vi "HFRR ADV v011 new software.vi"() -> ()   [LabVIEW 2025] (continued)
            n1484 = Equal?(x=w2429, y=10) -> (x = y?=w2427:bool)
            n1485 = case shown="True" w2427 {
              frame False {
                n1486 = property on="ENTER THE NEW PASSWORD" class="Str"("Visible"=FALSE) -> ()  [unwired: 2 in, 2 out]
              }
              frame True {
                # "password"
                # "change password logic"
                n1487 = local read "ENTER CURRENT PASSWORD"() -> (w2446:string)
                n1488 = local read "dipl pwd"() -> (w2440:string)
                n1489 = String To Byte Array(string=w2446) -> (unsigned byte array=w2448:u8[])
                n1490 = String To Byte Array(string=w2440) -> (unsigned byte array=w2441:u8[])
                n1491 = Array Size(array=w2448) -> (size(s)=w2445:i32)
                n1492 = Array Size(array=w2441) -> (size(s)=w2443:i32)
                n1493 = for {
                  N: w2445 -> [_]
                  tunnel: w2448 -> [w2472]
                  tunnel: [w2470] -> w2449 mode=indexing
                  tunnel: w2445 -> [w2464]
                  i -> [w2465]
                  n1494 = Decrement(x=w2464) -> (x-1=w2462:i32)
                  n1495 = Equal?(x=w2465, y=w2462) -> (x = y?=w2463:bool)
                  n1496 = Index Array(array=w2472, index=w2465) -> (element=w2466:u8)
                  n1497 = Number To Decimal String(number=w2466) -> (decimal integer string=w2471:string)  [unwired: 1 in]
                  n1498 = Select(t="", s=w2463, f="\r") -> (s? t:f=w2468:string)
                  n1499 = Concatenate Strings(w2471, w2468) -> (w2470:string)
                }
                n1500 = for {
                  N: w2443 -> [_]
                  tunnel: w2441 -> [w2460]
                  tunnel: [w2458] -> w2442 mode=indexing
                  tunnel: w2443 -> [w2455]
                  i -> [w2456]
                  n1501 = Decrement(x=w2455) -> (x-1=w2454:i32)
                  n1502 = Equal?(x=w2456, y=w2454) -> (x = y?=w2453:bool)
                  n1503 = Index Array(array=w2460, index=w2456) -> (element=w2459:u8)
                  n1504 = Number To Decimal String(number=w2459) -> (decimal integer string=w2457:string)  [unwired: 1 in]
                  n1505 = Select(t="", s=w2453, f="\r") -> (s? t:f=w2450:string)
                  n1506 = Concatenate Strings(w2457, w2450) -> (w2458:string)
                }
                n1507 = local read "string"() -> (w2447:string)
                n1508 = Concatenate Strings(w2442) -> (w2436:string)
                n1509 = Concatenate Strings(w2447) -> (w2444:string)
                n1510 = Concatenate Strings(w2449) -> (w2437:string)
                n1511 = Equal?(x=w2437, y=w2444) -> (x = y?=w2439:bool)
                n1512 = Equal?(x=w2437, y=w2436) -> (x = y?=w2435:bool)
                n1513 = Or(x=w2439, y=w2435) -> (x .or. y?=w2438:bool)
                n1514 = case shown="True" w2438 {
                  frame False {
                  }
                  frame True {
                    n1515 = property on="ENTER THE NEW PASSWORD" class="Str"("Visible"=TRUE) -> ()  [unwired: 2 in, 2 out]
                  }
                }
              }
            }
          }
          frame #2 {
            n1516 = String To Byte Array(string="ENTER THE NEW PASSWORD") -> (unsigned byte array=w2475:u8[])
            n1517 = Search 1D Array(1D array=w2475, element=u8 10) -> (index of element=w2479:i32)  [unwired: 1 in]
            n1518 = Index Array(array=w2475, index=w2479) -> (element=w2477:u8)
            n1519 = Equal?(x=w2477, y=10) -> (x = y?=w2474:bool)
            n1520 = case shown="False" w2474 {
              frame False {
              }
              frame True {
                n1521 = local write "EDIT"(FALSE) -> ()
                n1522 = local write "SrvM CP"(FALSE) -> ()
                n1523 = local read "ENTER THE NEW PASSWORD"() -> (w2482:string)
                n1524 = String To Byte Array(string=w2482) -> (unsigned byte array=w2487:u8[])
                n1525 = Array Size(array=w2487) -> (size(s)=w2484:i32)
                n1526 = for {
                  N: w2484 -> [_]
                  tunnel: w2487 -> [w2500]
                  tunnel: [w2497] -> w2489 mode=indexing
                  tunnel: w2484 -> [w2492]
                  i -> [w2490]
                  n1527 = Decrement(x=w2492) -> (x-1=w2493:i32)
                  n1528 = Equal?(x=w2490, y=w2493) -> (x = y?=w2494:bool)
                  n1529 = Index Array(array=w2500, index=w2490) -> (element=w2499:u8)
                  n1530 = Number To Decimal String(number=w2499) -> (decimal integer string=w2498:string)  [unwired: 1 in]
                  n1531 = Select(t="", s=w2494, f="\r") -> (s? t:f=w2491:string)
                  n1532 = Concatenate Strings(w2498, w2491) -> (w2497:string)
                }
                n1533 = local read "file path"() -> (w2481:path)
                n1534 = Concatenate Strings(w2489) -> (w2483:string)
                n1535 = Delete(path (use dialog)=w2481) -> (deleted path=w2485:path)  [unwired: 4 in, 2 out]
                n1536 = call <vilib>:"Write Characters To File.vi"("append to file? (new file:F)"=FALSE, "character string"=w2483, "file path (dialog if empty)"=w2485) -> ()  [unwired: 2 in, 1 out]
              }
            }
          }
          frame #3 {
            n1537 = case shown="True" "SrvM CP" {
              frame False {
                w2503 = ""
                n1538 = local write "ENTER CURRENT PASSWORD"(w2503) -> ()
                n1539 = local write "ENTER THE NEW PASSWORD"(w2503) -> ()
                n1540 = property on="ENTER CURRENT PASSWORD" class="Str"("Visible"=FALSE) -> ()  [unwired: 2 in, 2 out]
              }
              frame True {
                n1541 = property on="ENTER THE NEW PASSWORD" class="Str"() -> ("Visible"=w2504:bool)  [unwired: 2 in, 2 out]
                n1542 = Not(x=w2504) -> (.not. x?=w2505:bool)
                n1543 = property on="ENTER CURRENT PASSWORD" class="Str"("Visible"=w2505) -> ()  [unwired: 2 in, 2 out]
              }
            }
          }
          frame #4 {
            n1544 = String To Byte Array(string="Password") -> (unsigned byte array=w2512:u8[])
            n1545 = Search 1D Array(1D array=w2512, element=u8 10) -> (index of element=w2510:i32)  [unwired: 1 in]
            n1546 = Index Array(array=w2512, index=w2510) -> (element=w2511:u8)
            n1547 = Equal?(x=w2511, y=10) -> (x = y?=w2507:bool)
            n1548 = case shown="True" w2507 {
              frame False {
              }
              frame True {
                # "password"
                # "password"
                n1549 = local read "Password"() -> (w2525:string)
                n1550 = String To Byte Array(string=w2525) -> (unsigned byte array=w2528:u8[])
                n1551 = String To Byte Array(string="@143$\n") -> (unsigned byte array=w2514:u8[])
                n1552 = Array Size(array=w2528) -> (size(s)=w2523:i32)
                n1553 = Array Size(array=w2514) -> (size(s)=w2519:i32)
                n1554 = for {
                  N: w2523 -> [_]
                  tunnel: w2528 -> [w2562]
                  tunnel: [w2560] -> w2529 mode=indexing
                  tunnel: w2523 -> [w2557]
                  i -> [w2558]
                  n1555 = Decrement(x=w2557) -> (x-1=w2556:i32)
                  n1556 = Index Array(array=w2562, index=w2558) -> (element=w2561:u8)
                  n1557 = Equal?(x=w2558, y=w2556) -> (x = y?=w2555:bool)
                  n1558 = Number To Decimal String(number=w2561) -> (decimal integer string=w2559:string)  [unwired: 1 in]
                  n1559 = Select(t="", s=w2555, f="\r") -> (s? t:f=w2552:string)
                  n1560 = Concatenate Strings(w2559, w2552) -> (w2560:string)
                }
                n1561 = for {
                  N: w2519 -> [_]
                  tunnel: w2514 -> [w2573]
                  tunnel: [w2571] -> w2517 mode=indexing
                  tunnel: w2519 -> [w2568]
                  i -> [w2569]
                  n1562 = Decrement(x=w2568) -> (x-1=w2567:i32)
                  n1563 = Index Array(array=w2573, index=w2569) -> (element=w2572:u8)
                  n1564 = Equal?(x=w2569, y=w2567) -> (x = y?=w2566:bool)
                  n1565 = Number To Decimal String(number=w2572) -> (decimal integer string=w2570:string)  [unwired: 1 in]
                  n1566 = Select(t="", s=w2566, f="\r") -> (s? t:f=w2563:string)
                  n1567 = Concatenate Strings(w2570, w2563) -> (w2571:string)
                }
                n1568 = local read "file path"() -> (w2513:path)
                n1569 = call <vilib>:"Read Characters From File.vi"("file path (dialog if empty)"=w2513) -> ("character string"=w2527:string)  [unwired: 5 in, 3 out]
                "string" <- w2527
                n1570 = flat-sequence {
                  tunnel: [w2530] -> w2524
                  frame #0 {
                    w2530 = ""
                    n1571 = local write "Password"(w2530) -> ()
                  }
                }
                n1572 = Concatenate Strings(w2517) -> (w2518:string)
                n1573 = Concatenate Strings(w2527) -> (w2526:string)
                n1574 = Concatenate Strings(w2529) -> (w2521:string)
                n1575 = Equal?(x=w2521, y=w2526) -> (x = y?=w2516:bool)
                n1576 = Equal?(x=w2521, y=w2518) -> (x = y?=w2522:bool)
                n1577 = Or(x=w2516, y=w2522) -> (x .or. y?=w2515:bool)
                "x = y?" <- w2515
                n1578 = case shown="True" w2515 {
                  selector: w2515 -> [w2532 _]
                  tunnel: w2524 -> [_ _]
                  frame False {
                    n1579 = And(x=w2532, y=TRUE ("Visible")) -> (x .and. y?=w2533:bool)
                    n1580 = property on="message" class="Str"("Visible"=w2533) -> ()  [unwired: 2 in, 2 out]
                  }
                  frame True {
                    n1581 = control-ref of="This VI"() -> (w2544:refnum<vi>)
                    n1582 = property class="VI"(reference=w2544) -> (reference out=w2535:refnum<vi>, error out=w2539:errorcluster, "Panel"=w2543:refnum<vi>)  [unwired: 1 in]
                    n1583 = property on="message" class="Str"("Visible"=FALSE) -> ()  [unwired: 2 in, 2 out]
                    n1584 = property class="Pnl"(reference=w2543, error in=w2539) -> (reference out=w2537:refnum<vi>, error out=w2540:errorcluster, "Panes[]"=w2542:refnum<vi>[])
                    n1585 = for {
                      tunnel: w2542 -> [w2551] mode=indexing
                      tunnel: T20."Always On" ("Horizontal Scrollbar Visibility") -> [w2550]
                      tunnel: w2540 -> [w2547]
                      tunnel: [w2546] -> w2538
                      n1586 = property class="Pane"(reference=w2551, error in=w2547, "HorizScrollbarVisibility"=w2550) -> (reference out=w2548:refnum<vi>, error out=w2549:errorcluster)
                      n1587 = Close Reference(reference=w2548, error in (no error)=w2549) -> (error out=w2546:errorcluster)
                    }
                    n1588 = Close Reference(reference=w2537, error in (no error)=w2538) -> (error out=w2536:errorcluster)
                    n1589 = Close Reference(reference=w2535, error in (no error)=w2536) -> (error out=→"error out 6":errorcluster)
                  }
                }
              }
            }
          }
        }
        n1590 = local read "x = y?"() -> (w2372:bool)
        n1591 = local read "HUMIDITY: 2"() -> (w2374:dbl)
        n1592 = local read "HUMIDITY:"() -> (w2373:dbl)
        n1593 = property on="Port 2 Error" class="Clust (strict)"("Visible"="EDIT") -> ()  [unwired: 2 in, 2 out]
        n1594 = property on="Port 1 Error" class="Clust (strict)"("Visible"="EDIT") -> ()  [unwired: 2 in, 2 out]
        n1595 = case shown="True" "SrvM CP 2" {
          frame False {
          }
          frame True {
            n1596 = local write "SrvM CP 2"(FALSE ("SrvM CP 2")) -> ()
            n1597 = local read "HUMIDITY: 2"() -> (w2413:dbl)
            n1598 = local read "TEMP INTERCEPT: 2"() -> (w2412:dbl)
            n1599 = local read "DISPLACEMENT : 4"() -> (w2416:dbl)
            n1600 = local read "TEMPERATURE : 2"() -> (w2415:dbl)
            n1601 = local read "STROKE GAIN : 2"() -> (w2417:dbl)
            n1602 = local read "FRIC. FORCE : 2"() -> (w2418:dbl)
            n1603 = local read "AIR TEMP INTERCEPT: 2"() -> (w2411:dbl)
            n1604 = local read "AIR TEMPERATURE : 2"() -> (w2414:dbl)
            n1605 = local write "HUMIDITY:"(w2413) -> ()
            n1606 = local write "AIR TEMP INTERCEPT:"(w2412) -> ()
            n1607 = local write "TEMPERATURE :"(w2415) -> ()
            n1608 = local write "FRIC. FORCE :"(w2418) -> ()
            n1609 = local write "STROKE GAIN :"(w2417) -> ()
            n1610 = local write "DISPLACEMENT :"(w2416) -> ()
            n1611 = local write "AIR TEMPERATURE :"(w2414) -> ()
            n1612 = local write "TEMP INTERCEPT:"(w2411) -> ()
          }
        }
        n1613 = Or(x="SAVE", y=w2366) -> (x .or. y?=w2367:bool)
        n1614 = And(x="EDIT", y=w2372) -> (x .and. y?=w2370:bool)
        n1615 = local read "DISPLACEMENT : 4"() -> (w2383:dbl)
        n1616 = local read "TEMPERATURE : 2"() -> (w2381:dbl)
        n1617 = local read "STROKE GAIN : 2"() -> (w2387:dbl)
        n1618 = local read "DISPLACEMENT :"() -> (w2382:dbl)
        n1619 = local read "FRIC. FORCE : 2"() -> (w2390:dbl)
        n1620 = local read "TEMPERATURE :"() -> (w2379:dbl)
        n1621 = local read "STROKE GAIN :"() -> (w2386:dbl)
        n1622 = local read "FRIC. FORCE :"() -> (w2389:dbl)
        n1623 = case shown="True" w2370 {
          tunnel: [u8 2 ("Disabled") u8 0 ("Disabled")] -> w2369
          tunnel: [w2734 TRUE ("Visible")] -> w2368
          frame False {
            w2734 = FALSE ("Visible")
            n1624 = local write "EDIT 2"(w2734) -> ()
          }
          frame True {
          }
        }
        n1625 = case shown="True" w2367 {
          frame False {
          }
          frame True {
            n1626 = stacked-sequence {
              seq-local: [w2582 _ _] -> [_ w2729 _]
              frame #0 {
                (unwired) i16 5 ("precision (6)")
                # "[CH1]    - FF\n[CH2]   - TEMPERATURE\n[CH3]    - Humidity\n[CH4]    - AIR TEMP\n[CH5]\\- Visa Uno\n[CH6] \\- Visa Due\n[CH7]  \\- file path\n[CH8]   - Displacement Gain\n[CHA]   - Stroke Gain\n[CHB]   - Stroke PID Gain\n[CHC]   -Language Selection\n[CHD]   -Power +\n[CHE]   -Power_\n[CHF]   -Heater\n[CHG]   -Humidity Wet\n[CHH]   -Humidity Dry\n[CHI]   -Integral Time"
                n1627 = local read "Language Selection"() -> (w2630:enum16{"English", "Russian"})
                n1628 = local read "CH-HUMIDITY WET"() -> (w2588:u16)
                n1629 = local read "CH-HUMIDITY DRY"() -> (w2585:u16)
                n1630 = local read "STROKE GAIN :"() -> (w2574:dbl)
                n1631 = local read "CH-POWER +"() -> (w2597:u16)
                n1632 = local read "CH-POWER -"() -> (w2594:u16)
                n1633 = local read "CH-HEATER"() -> (w2591:u16)
                n1634 = local read "AIR TEMPERATURE :"() -> (w2577:dbl)
                n1635 = local read "DISPLACEMENT :"() -> (w2575:dbl)
                n1636 = local read "TEMPERATURE :"() -> (w2578:dbl)
                n1637 = local read "FRIC. FORCE :"() -> (w2579:dbl)
                n1638 = local read "HUMIDITY:"() -> (w2576:dbl)
                n1639 = Path To String(path="File Path") -> (string=w2646:string)
                n1640 = Number To Fractional String(number=w2574, width (-)=i16 10 ("precision (6)"), precision (6)=i16 5) -> (F-format string=w2637:string)  [unwired: 1 in]
                n1641 = Number To Fractional String(number=w2630, width (-)=i16 10 ("precision (6)"), precision (6)=i16 5) -> (F-format string=w2626:string)  [unwired: 1 in]
                n1642 = Number To Fractional String(number=w2597, width (-)=i16 10 ("precision (6)"), precision (6)=i16 5) -> (F-format string=w2620:string)  [unwired: 1 in]
                n1643 = Number To Fractional String(number=w2594, width (-)=i16 10 ("precision (6)"), precision (6)=i16 5) -> (F-format string=w2617:string)  [unwired: 1 in]
                n1644 = Number To Fractional String(number=w2591, width (-)=i16 10 ("precision (6)"), precision (6)=i16 5) -> (F-format string=w2612:string)  [unwired: 1 in]
                n1645 = Number To Fractional String(number=w2588, width (-)=i16 10 ("precision (6)"), precision (6)=i16 5) -> (F-format string=w2609:string)  [unwired: 1 in]
                n1646 = Number To Fractional String(number=w2585, width (-)=i16 10 ("precision (6)"), precision (6)=i16 5) -> (F-format string=w2604:string)  [unwired: 1 in]
                n1647 = local read "Com Port 1"() -> (w2581:refnum<visa-resource-name>)
                n1648 = local read "Com Port 2"() -> (w2580:refnum<visa-resource-name>)
                n1649 = Concatenate Strings(w2646, "\\" ("string")) -> (w2645:string)
                n1650 = Number To Fractional String(number=w2579, width (-)=i16 10 ("precision (6)"), precision (6)=i16 5) -> (F-format string=w2678:string)  [unwired: 1 in]
                n1651 = Number To Fractional String(number=w2578, width (-)=i16 10 ("precision (6)"), precision (6)=i16 5) -> (F-format string=w2677:string)  [unwired: 1 in]
                n1652 = Number To Fractional String(number=w2576, width (-)=i16 10 ("precision (6)"), precision (6)=i16 5) -> (F-format string=w2671:string)  [unwired: 1 in]
                n1653 = Number To Fractional String(number=w2577, width (-)=i16 10 ("precision (6)"), precision (6)=i16 5) -> (F-format string=w2665:string)  [unwired: 1 in]
                n1654 = Number To Fractional String(number=w2575, width (-)=i16 10 ("precision (6)"), precision (6)=i16 5) -> (F-format string=w2638:string)  [unwired: 1 in]
                n1655 = Concatenate Strings("[CHA]" ("string"), w2637, "- Stroke Gain" ("string"), "\r") -> (w2631:string)
                n1656 = Concatenate Strings("[CHC]" ("string"), w2626, "-Language Selection" ("string"), "\r") -> (w2623:string)
                n1657 = Concatenate Strings("[CHD]" ("string"), w2620, "-Power +" ("string"), "\r") -> (w2602:string)
                n1658 = Concatenate Strings("[CHG]" ("string"), w2609, "-Humidity Wet" ("string"), "\r") -> (w2599:string)
                n1659 = Concatenate Strings("[CHH]" ("string"), w2604, "-Humidity Dry" ("string"), "\r") -> (w2598:string)
                n1660 = Concatenate Strings("[CH1]" ("string"), w2678, " - FF" ("string"), "\r") -> (w2676:string)
                n1661 = Concatenate Strings("[CH2]" ("string"), w2677, " - TEMPERATURE" ("string"), "\r") -> (w2675:string)
                n1662 = Concatenate Strings("[CH3]" ("string"), w2671, " - Humidity" ("string"), "\r") -> (w2668:string)
                n1663 = Concatenate Strings("[CH4]" ("string"), w2665, " - AIR TEMP" ("string"), "\r") -> (w2661:string)
                n1664 = Concatenate Strings("[CH5]" ("string"), w2581, "- Visa Uno" ("string"), "\r") -> (w2654:string)
                n1665 = Concatenate Strings("[CH6]" ("string"), w2580, "- Visa Due" ("string"), "\r") -> (w2649:string)
                n1666 = Concatenate Strings("[CH7]" ("string"), w2645, "- file path" ("string"), "\r") -> (w2648:string)
                n1667 = Concatenate Strings("[CH8]" ("string"), w2638, "- Displacement Gain" ("string"), "\r") -> (w2641:string)
                n1668 = Concatenate Strings("[CHE]" ("string"), w2617, "-Power_" ("string"), "\r") -> (w2601:string)
                n1669 = Concatenate Strings("[CHF]" ("string"), w2612, "-Heater" ("string"), "\r") -> (w2600:string)
                n1670 = Concatenate Strings(w2676, w2675, w2668, w2661, w2654, w2649, w2648, w2641, w2631, w2623, w2602, w2601, w2600, w2599, w2598) -> (w2582:string)
                "gain" <- w2582
              }
              frame #1 {
                n1671 = local read "Camera Port :"() -> (w2690:string)
                n1672 = local read "C3 :"() -> (w2698:refnum<visa-resource-name>)
                n1673 = local read "TEMP INTERCEPT:"() -> (w2699:dbl)
                n1674 = local read "AIR TEMP INTERCEPT:"() -> (w2700:dbl)
                n1675 = local read "Com Port 3"() -> (w2701:refnum<visa-resource-name>)
                n1676 = Concatenate Strings("[CH8]" ("string"), w2690, "- Visa Camera" ("string"), "\r") -> (w2689:string)
                n1677 = Concatenate Strings("[CH7]" ("string"), w2698, "- Visa Humidity" ("string"), "\r") -> (w2694:string)
                n1678 = Number To Fractional String(number=w2699, width (-)=i16 10 ("precision (6)"), precision (6)=i16 5) -> (F-format string=w2717:string)  [unwired: 1 in]
                n1679 = Concatenate Strings("[CHL]" ("string"), w2701, "- Visa humid" ("string"), "\r") -> (w2704:string)
                n1680 = Number To Fractional String(number=w2700, width (-)=i16 10 ("precision (6)"), precision (6)=i16 5) -> (F-format string=w2724:string)  [unwired: 1 in]
                n1681 = Concatenate Strings("[CHK]" ("string"), w2717, "-TEMP INTERCEPT" ("string"), "\r") -> (w2713:string)
                n1682 = Concatenate Strings("[SNO]" ("string"), "S.NO", "-" ("string"), "\r") -> (w2709:string)
                n1683 = Concatenate Strings("[CHJ]" ("string"), w2724, "-AIR TEMP INTERCEPT" ("string"), "\r") -> (w2714:string)
                n1684 = String To Path(string="C:\\LAB-IQ\\calibrate WO 2465.dcf") -> (path=w2702:path)
                n1685 = Concatenate Strings(w2729, w2714, w2713, w2709, w2704, w2694, w2689) -> (w2728:string)
                n1686 = call <vilib>:"Write Characters To File.vi"("append to file? (new file:F)"=FALSE, "character string"=w2728, "file path (dialog if empty)"=w2702) -> ()  [unwired: 2 in, 1 out]
              }
              frame #2 {
                n1687 = local write "Lan flag"(0.0 ("Lan flag")) -> ()
                n1688 = local write "conststatus"(0.0 ("rpm value : 2")) -> ()
                n1689 = local write "SAVE"(FALSE ("OK Button 14")) -> ()
                n1690 = local write "SAVE 2"(FALSE ("SAVE 2")) -> ()
              }
            }
          }
        }
        n1691 = Subtract(x=w2374, y=w2373) -> (x-y=w2375:dbl)
        n1692 = local read "AIR TEMPERATURE : 2"() -> (w2378:dbl)
        n1693 = local read "AIR TEMPERATURE :"() -> (w2377:dbl)
        n1694 = Divide(x=w2375, y=w2373) -> (x/y=w2397:dbl)
        n1695 = Subtract(x=w2390, y=w2389) -> (x-y=w2388:dbl)
        n1696 = Subtract(x=w2381, y=w2379) -> (x-y=w2380:dbl)
        n1697 = Subtract(x=w2387, y=w2386) -> (x-y=w2385:dbl)
        n1698 = Subtract(x=w2383, y=w2382) -> (x-y=w2384:dbl)
        n1699 = Subtract(x=w2378, y=w2377) -> (x-y=w2376:dbl)
        n1700 = Divide(x=w2388, y=w2389) -> (x/y=w2408:dbl)
        n1701 = Divide(x=w2380, y=w2379) -> (x/y=w2401:dbl)
        n1702 = Divide(x=w2385, y=w2386) -> (x/y=w2405:dbl)
        n1703 = Divide(x=w2384, y=w2382) -> (x/y=w2404:dbl)
        n1704 = Multiply(x=w2397, y=100.0) -> (x*y=→"HUMIDITY  Calibration Error":dbl)
        n1705 = Divide(x=w2376, y=w2377) -> (x/y=w2400:dbl)
        n1706 = Multiply(x=w2408, y=100.0) -> (x*y=→"FRIC. FORCE Calibration Error":dbl)
        n1707 = Multiply(x=w2401, y=100.0) -> (x*y=→"TEMPERATURE  Calibration Error":dbl)
        n1708 = Multiply(x=w2405, y=100.0) -> (x*y=→"STROKE Calibration Error":dbl)
        n1709 = Multiply(x=w2404, y=100.0) -> (x*y=→"DISPLACEMENT  Calibration Error":dbl)
        n1710 = property on="EDIT 2" class="Bool (strict)"("Visible"=w2368) -> ()  [unwired: 2 in, 2 out]
        n1711 = property on="SAVE" class="Bool (strict)"("Visible"=w2368) -> ()  [unwired: 2 in, 2 out]
        n1712 = property on="SrvM CP" class="Bool (strict)"("Disabled"=w2369) -> ()  [unwired: 2 in, 2 out]
        n1713 = property on="visa due" class="CmbBox"("Disabled"=w2369) -> ()  [unwired: 2 in, 2 out]
        n1714 = property on="File Path" class="Path"("Disabled"=w2369) -> ()  [unwired: 2 in, 2 out]
        n1715 = Multiply(x=w2400, y=100.0) -> (x*y=→"AIR TEMPERATURE  Calibration Error":dbl)
        n1716 = property on="Language Selection" class="Enum (strict)"("Visible"=w2368) -> ()  [unwired: 2 in, 2 out]
        n1717 = property on="Tab Control 7" class="TabCtl (strict)"("Disabled"=w2369) -> ()  [unwired: 2 in, 2 out]
        n1718 = property on="AIR TEMP INTERCEPT:" class="DigNum (strict)"("Disabled"=w2369) -> ()  [unwired: 2 in, 2 out]
        n1719 = property on="CH-POWER -" class="DigNum (strict)"("Disabled"=w2369) -> ()  [unwired: 2 in, 2 out]
        n1720 = property on="CH-POWER +" class="DigNum (strict)"("Disabled"=w2369) -> ()  [unwired: 2 in, 2 out]
        n1721 = property on="AIR TEMPERATURE :" class="DigNum (strict)"("Disabled"=w2369) -> ()  [unwired: 2 in, 2 out]
        n1722 = property on="STROKE GAIN :" class="DigNum (strict)"("Disabled"=w2369) -> ()  [unwired: 2 in, 2 out]
        n1723 = property on="SPEED OUT:" class="DigNum (strict)"("Disabled"=w2369) -> ()  [unwired: 2 in, 2 out]
        n1724 = property on="CH-HUMIDITY DRY" class="DigNum (strict)"("Disabled"=w2369) -> ()  [unwired: 2 in, 2 out]
        n1725 = property on="HUMIDITY:" class="DigNum (strict)"("Disabled"=w2369) -> ()  [unwired: 2 in, 2 out]
        n1726 = property on="CH-HUMIDITY WET" class="DigNum (strict)"("Disabled"=w2369) -> ()  [unwired: 2 in, 2 out]
        n1727 = property on="TEMPERATURE :" class="DigNum (strict)"("Disabled"=w2369) -> ()  [unwired: 2 in, 2 out]
        n1728 = property on="DISPLACEMENT :" class="DigNum (strict)"("Disabled"=w2369) -> ()  [unwired: 2 in, 2 out]
        n1729 = property on="CH-HEATER" class="DigNum (strict)"("Disabled"=w2369) -> ()  [unwired: 2 in, 2 out]
        n1730 = property on="TEMP INTERCEPT:" class="DigNum (strict)"("Disabled"=w2369) -> ()  [unwired: 2 in, 2 out]
        n1731 = property on="FRIC. FORCE :" class="DigNum (strict)"("Disabled"=w2369) -> ()  [unwired: 2 in, 2 out]
      }
    }
    n1732 = local read "RUN"() -> (w1763:bool)
    n1733 = local read "RUN"() -> (w1761:bool)
    n1734 = disable-structure shown="Disabled" {
      disable-tunnel: [w1778 _] -> w1744
      disable-tunnel: [w1777 _] -> w1742
      frame Disabled {
        n1735 = local read "Temperature before test"() -> (w1771:dbl)
        n1736 = local read "Temperature after test"() -> (w1784:dbl)
        n1737 = case shown="True" "Save Results" {
          frame False {
          }
          frame True {
            w1800 = "\r"
            n1738 = local write "Save Results"(FALSE ("OK Button 5")) -> ()
            n1739 = local read "Temperature before test"() -> (w1838:dbl)
            n1740 = local read "Temperature after test"() -> (w1840:dbl)
            n1741 = local read "Humidity before test"() -> (w1837:dbl)
            n1742 = local read "Humidity after test"() -> (w1839:dbl)
            n1743 = local read "WS1.4"() -> (w1844:dbl)
            n1744 = local read "AVP"() -> (w1842:dbl)
            n1745 = Number To Fractional String(number=w1844, width (-)=i16 6, precision (6)=i16 1) -> (F-format string=w1804:string)  [unwired: 1 in]
            n1746 = local read "MWSD"() -> (w1841:dbl)
            n1747 = local read "String"() -> (w1833:string)
            n1748 = local read "FILE"() -> (w1836:string)
            n1749 = local read "HCF"() -> (w1843:dbl)
            n1750 = Number To Fractional String(number=w1837, width (-)=i16 6, precision (6)=i16 1) -> (F-format string=w1829:string)  [unwired: 1 in]
            n1751 = Number To Fractional String(number=w1838, width (-)=i16 6, precision (6)=i16 1) -> (F-format string=w1826:string)  [unwired: 1 in]
            n1752 = Number To Fractional String(number=w1839, width (-)=i16 6, precision (6)=i16 1) -> (F-format string=w1822:string)  [unwired: 1 in]
            n1753 = Number To Fractional String(number=w1840, width (-)=i16 6, precision (6)=i16 1) -> (F-format string=w1818:string)  [unwired: 1 in]
            n1754 = Number To Fractional String(number=w1842, width (-)=i16 6, precision (6)=i16 3) -> (F-format string=w1811:string)  [unwired: 1 in]
            n1755 = Concatenate Strings(w1833, w1836) -> (w1855:string)
            n1756 = Number To Fractional String(number=w1841, width (-)=i16 6, precision (6)=i16 1) -> (F-format string=w1815:string)  [unwired: 1 in]
            n1757 = Number To Fractional String(number=w1843, width (-)=i16 6, precision (6)=i16 2) -> (F-format string=w1809:string)  [unwired: 1 in]
            n1758 = Concatenate Strings("(" ("string"), w1804, ")Microns" ("string")) -> (w1803:string)
            n1759 = local read "REMARKS"() -> (w1835:string)
            "REMARKS 2" <- w1835
            n1760 = Concatenate Strings("(" ("string"), w1829, " ) % RH," ("string")) -> (w1830:string)
            n1761 = Concatenate Strings(w1809, ")" ("string")) -> (w1807:string)
            n1762 = Concatenate Strings("(" ("string"), w1826, ")  Deg C ," ("string")) -> (w1825:string)
            n1763 = Concatenate Strings("(" ("string"), w1822, " ) % RH," ("string")) -> (w1821:string)
            n1764 = Concatenate Strings("(" ("string"), w1818, ")  Deg C ," ("string")) -> (w1817:string)
            n1765 = Concatenate Strings("(" ("string"), w1815, ")  Microns," ("string")) -> (w1814:string)
            n1766 = Concatenate Strings("(" ("string"), w1811, ")  kPa," ("string")) -> (w1801:string)
            n1767 = Concatenate Strings(w1855, ".dwm" ("Substring")) -> (w1853:string)
            n1768 = String To Path(string=w1853) -> (path=w1852:path)
            n1769 = Concatenate Strings(w1835, w1800, " Humidity before test= " ("Substring"), w1830, w1800, " Temperature before test = " ("Substring"), w1825, w1800, " Humidity after test= " ("Substring"), w1821, w1800, "Temperature after test = " ("Substring"), w1817, w1800, "MSD = " ("Substring"), w1814, w1800, "  AVP = " ("Substring"), w1801, w1800, "  HCF                     =( " ("Substring"), w1807, w1800, " WS1.4                  = " ("Substring"), w1803, w1800) -> (w1799:string)
            "data" <- w1799
            n1770 = call <vilib>:"Write Characters To File.vi"("append to file? (new file:F)"=FALSE, "character string"=w1799, "file path (dialog if empty)"=w1852) -> ()  [unwired: 2 in, 1 out]
            n1771 = Match Pattern(string=w1799, regular expression="!") -> (after substring=→"export":string)  [unwired: 1 in, 3 out]
          }
        }
        n1772 = Add(x=231.864, y=w1771) -> (x+y=w1768:dbl)
        n1773 = Add(x=231.864, y=w1784) -> (x+y=w1781:dbl)
        n1774 = Divide(x=1705.984, y=w1768) -> (x/y=w1769:dbl)
        n1775 = Divide(x=1705.984, y=w1781) -> (x/y=w1782:dbl)
        n1776 = local read "Humidity before test"() -> (w1773:dbl)
        n1777 = local read "Humidity after test"() -> (w1786:dbl)
        n1778 = Subtract(x=8.017352 ("y"), y=w1769) -> (x-y=w1795:dbl)
        n1779 = Subtract(x=8.017352 ("y"), y=w1782) -> (x-y=w1789:dbl)
        n1780 = expression code="10**y"(w1795) -> (w1775:dbl)
        n1781 = expression code="10**y"(w1789) -> (w1788:dbl)
        n1782 = Multiply(x=w1773, y=w1775) -> (x*y=w1774:dbl)
        n1783 = Multiply(x=w1786, y=w1788) -> (x*y=w1787:dbl)
        n1784 = Divide(x=w1774, y=750.0) -> (x/y=w1790:dbl)
        n1785 = Divide(x=w1787, y=750.0) -> (x/y=w1791:dbl)
        n1786 = Add(x=w1790, y=w1791) -> (x+y=w1792:dbl)
        n1787 = Divide(x=w1792, y=2.0) -> (x/y=w1794:dbl)
        n1788 = local write "AVP"(w1794) -> ()
        n1789 = Subtract(x=1.4, y=w1794) -> (x-y=w1777:dbl)
        n1790 = local read "HCF"() -> (w1778:dbl)
      }
      frame Enabled {
      }
    }
    n1791 = case shown="True" "EDIT 3" {
      frame False {
      }
      frame True {
        n1792 = local write "EDIT 3"(FALSE ("EDIT 3")) -> ()
        n1793 = local write "Main Tab"(T2."About" ("Main Tab")) -> ()
      }
    }
    n1794 = case shown="False" w1763 {
      frame False {
        n1795 = local read "stopT"() -> (w2741:bool)
        n1796 = case shown="True" w2741 {
          frame False {
          }
          frame True {
            n1797 = local write "stopT"(FALSE) -> ()
          }
        }
      }
      frame True {
        "stopT" <- TRUE
      }
    }
    n1798 = case shown="False" w1761 {
      frame False {
      }
      frame True {
      }
    }
    n1799 = case shown="True" w1751 {
      frame False {
        n1800 = property on="Password 2" class="Str"("Visible"=FALSE) -> ()  [unwired: 2 in, 2 out]
        n1801 = local write "Password 2"("" ("Password")) -> ()
      }
      frame True {
        n1802 = property on="Password 2" class="Str"("Visible"=TRUE) -> ()  [unwired: 2 in, 2 out]
        n1803 = Equal?(x="Password 2", y="HFRR1234") -> (x = y?=w1883:bool)
        n1804 = case shown="True" w1883 {
          tunnel: "Password 2" -> [w1886 _]
          frame False {
            n1805 = String Length(string=w1886) -> (length=w1887:i32)
            n1806 = Greater Than 0?(x=w1887) -> (x > 0?=w1885:bool)
            n1807 = case shown="False" w1885 {
              frame False {
                n1808 = property on="Password 2" class="Str"("Caption.Text"="Password (Advance Setting)") -> ()  [unwired: 2 in, 2 out]
              }
              frame True {
                n1809 = property on="Password 2" class="Str"("Caption.Text"="Incorrect Password!") -> ()  [unwired: 2 in, 2 out]
              }
            }
          }
          frame True {
            n1810 = local write "EDIT 2"(FALSE ("EDIT 2")) -> ()
            n1811 = local write "Password 2"("" ("Password")) -> ()
            n1812 = local write "Main Tab"(T2."Advance" ("Main Tab")) -> ()
            n1813 = local write "Main Dashboard Buttons"(T1."Advance" ("Main Dashboard Buttons")) -> ()
          }
        }
      }
    }
    n1814 = case shown="True" "Prog Uno" {
      frame False {
      }
      frame True {
        n1815 = stacked-sequence {
          frame #0 {
            n1816 = Delete(path (use dialog)=path "C:/LAB-IQ-NXT/UNOCOMPILE.bat" ("working directory")) -> ()  [unwired: 4 in, 3 out]
          }
          frame #1 {
            n1817 = local read "Com Port 1"() -> (w2348:refnum<visa-resource-name>)
            n1818 = Concatenate Strings("cmd.exe /c \"mode " ("command line"), w2348, ":1200,n,8,1\"\n" ("command line")) -> (w2353:string)
            n1819 = Concatenate Strings(w2353, "CD\\\nCD WinDucom\navrdude -C avrdude.conf -v -patmega328p -carduino -P" ("command line"), w2348, " -b115200 -D -Uflash:w:UNO_V20.hex:i\n" ("command line"), "\r") -> (w2355:string)
            "STR" <- w2355
            n1820 = call <vilib>:"Write Characters To File.vi"("append to file? (new file:F)"=FALSE, "character string"=w2355, "file path (dialog if empty)"=path "C:/LAB-IQ/UNOCOMPILE.bat" ("working directory")) -> ()  [unwired: 2 in, 1 out]
          }
          frame #2 {
            n1821 = disable-structure shown="Disabled" {
              frame Disabled {
                w2359 = "cmd.exe  /c \"C:\\LAB-IQ-NXT\\UNOCOMPILE.bat\"" ("string")
                n1822 = local write "Prog Uno"(FALSE ("run minimized? (F)")) -> ()
                n1823 = call <vilib>:"System Exec.vi"("expected output size  (4096)"=u32 65535, "run minimized? (F)"=FALSE, "wait until completion? (T)"=TRUE ("run minimized? (F)"), "working directory"=path "C:/LAB-IQ-NXT", "standard input"=w2359, "command line"=w2359) -> ("error out"=w2358:errorcluster, "standard output"=→"String 42":string)  [unwired: 2 in, 2 out]
                "error out 3" <- w2358
                n1824 = flat-sequence {
                  tunnel: w2358 -> [_]
                  frame #0 {
                  }
                }
              }
              frame Enabled {
              }
            }
          }
        }
      }
    }
    n1825 = case shown="\"ISO 12156\"" "TEST STANDARD" {
      tunnel: [2.0 ("Set Temp") 0.0 ("Set Temp") 2.0 ("Set Temp") 0.0 ("Set Temp")] -> w1752
      frame "ASTM D6079", Default {
        w2305 = 50.0 ("Hz")
        w2306 = 53.0 ("Set Rh")
        w2308 = 1.0 ("Set Strk")
        w2307 = 60.0 ("Set Temp")
        # "astm hide"
        n1826 = local write "NORMAL LOAD"(200.0 ("NORMAL LOAD")) -> ()
        n1827 = local write "Set Strk"(w2308) -> ()
        n1828 = local write "Set Hz"(w2305) -> ()
        n1829 = local write "Set Temp"(w2307) -> ()
        n1830 = local write "Set Rh"(w2306) -> ()
        n1831 = local write "test time"(75.0 ("test time")) -> ()
        n1832 = local write "Set Stroke:"(w2308) -> ()
        n1833 = local write "Set Humidity:"(w2306) -> ()
        n1834 = local write "Set Frequency:"(w2305) -> ()
        n1835 = local write "Set Temperature:"(w2307) -> ()
        "Test Standard" <- "ASTM D6079" ("Test Standard 2")
      }
      frame "ISO 12156" {
        n1836 = local write "Set Strk"(1.0 ("Set Strk")) -> ()
        n1837 = local write "NORMAL LOAD"(200.0 ("NORMAL LOAD")) -> ()
        n1838 = local write "Set Temp"(60.0 ("Set Temp")) -> ()
        n1839 = local write "test time"(75.0 ("test time")) -> ()
        n1840 = local write "Set Hz"(50.0 ("Hz")) -> ()
        n1841 = local write "Set Rh"(53.0 ("Set Rh")) -> ()
      }
      frame "CEC F-096-A-06" {
        n1842 = local write "Set Strk"(1.0 ("Set Strk")) -> ()
        n1843 = local write "NORMAL LOAD"(200.0 ("NORMAL LOAD")) -> ()
        n1844 = local write "Set Temp"(60.0 ("Set Temp")) -> ()
        n1845 = local write "test time"(75.0 ("test time")) -> ()
        n1846 = local write "Set Hz"(50.0 ("Hz")) -> ()
        n1847 = local write "Set Rh"(53.0 ("Set Rh")) -> ()
      }
      frame "Custom" {
      }
    }
    n1848 = case shown="True" "Prog Due" {
      frame False {
      }
      frame True {
        n1849 = stacked-sequence {
          frame #0 {
            n1850 = Delete(path (use dialog)=path "C:/LAB-IQ/DUECOMPILE.bat" ("working directory")) -> ()  [unwired: 4 in, 3 out]
          }
          frame #1 {
            n1851 = disable-structure shown="Disabled" {
              frame Disabled {
                n1852 = local read "visa due"() -> (w2330:string)
                n1853 = Concatenate Strings("cmd.exe /c \"mode " ("command line"), w2330, ":1200,n,8,1\"\n" ("command line")) -> (w2335:string)
                n1854 = Concatenate Strings(w2335, "CD\\\nCD WinDucom\nTIMEOUT 1\n bossac.exe -i -d --port=" ("command line"), w2330, " -U false -e -w -v -b DUE.bin -R\n" ("command line"), "\r") -> (w2337:string)
                "concatenated string 2" <- w2337
                n1855 = call <vilib>:"Write Characters To File.vi"("append to file? (new file:F)"=FALSE, "character string"=w2337, "file path (dialog if empty)"=path "C:/LAB-IQ-NXT/DUECOMPILE.bat" ("working directory")) -> ()  [unwired: 2 in, 1 out]
              }
              frame Enabled {
              }
            }
          }
          frame #2 {
            # "C:\\LAB-IQ-NXT\\DUECOMPILE.bat"
            n1856 = disable-structure shown="Disabled" {
              frame Disabled {
                w2342 = "cmd.exe  /c \"C:\\LAB-IQ-NXT\\DUECOMPILE.bat\"" ("string")
                n1857 = call <vilib>:"System Exec.vi"("expected output size  (4096)"=u32 65535, "run minimized? (F)"=FALSE, "wait until completion? (T)"=TRUE ("run minimized? (F)"), "working directory"=path "C:/LAB-IQ-NXT", "standard input"=w2342, "command line"=w2342) -> ("error out"=w2341:errorcluster, "standard output"=→"String 44":string)  [unwired: 2 in, 2 out]
                "error out 4" <- w2341
                n1858 = flat-sequence {
                  tunnel: w2341 -> [_]
                  frame #0 {
                  }
                }
              }
              frame Enabled {
              }
            }
            n1859 = local write "Prog Due"(FALSE ("Prog Due")) -> ()
          }
        }
      }
    }
    n1860 = Or(x=w1749, y=w1747) -> (x .or. y?=w1748:bool)
    n1861 = case shown="\"About\"" w1746 {
      tunnel: [T26."Acquire" ("Main Tab") T26."Compare Files" ("Main Tab") T26."About" ("Main Tab")] -> w1759
      frame "Acquire", Default {
      }
      frame "Compare Files" {
      }
      frame "About" {
      }
    }
    n1862 = Or(x=w1753, y="OPEN") -> (x .or. y?=w1754:bool)
    n1863 = case shown="True" w1754 {
      tunnel: w1753 -> [_ w1894]
      frame False {
      }
      frame True {
        n1864 = stacked-sequence {
          tunnel: w1894 -> [_ w1961 _ _]
          frame #0 {
            w1910 = "  " ("String 6")
            n1865 = local write "OPEN"(FALSE ("open")) -> ()
            n1866 = local read "string1 2"() -> (w1898:string)
            n1867 = local read "string1 3"() -> (w1897:string)
            n1868 = local read "string1 4"() -> (w1896:string)
            n1869 = property on="OPEN" class="Bool (strict)"("Visible"=FALSE) -> ()  [unwired: 2 in, 2 out]
            n1870 = local write "String 6"(w1910) -> ()
            n1871 = local write "String 7"(w1910) -> ()
            n1872 = local write "String 8"(w1910) -> ()
            n1873 = local write "String 12"(w1910) -> ()
            n1874 = local read "OK Button 16"() -> (w1895:bool)
            n1875 = String To Path(string=w1898) -> (path=w1906:path)
            n1876 = String To Path(string=w1897) -> (path=w1905:path)
            n1877 = String To Path(string=w1896) -> (path=w1904:path)
            n1878 = case shown="True" w1895 {
              tunnel: [w1911 w1912] -> w1899
              frame False {
                n1879 = local read "string1"() -> (w1911:string)
              }
              frame True {
                n1880 = local read "String Indicator 4"() -> (w1912:string)
              }
            }
            n1881 = Open/Create/Replace File "Open File"(file path (use dialog)=w1906) -> (refnum out=w1902:refnum<file>)  [unwired: 5 in, 2 out]
            n1882 = Open/Create/Replace File "Open File"(file path (use dialog)=w1905) -> (refnum out=w1901:refnum<file>)  [unwired: 5 in, 2 out]
            n1883 = Open/Create/Replace File "Open File"(file path (use dialog)=w1904) -> (refnum out=w1900:refnum<file>)  [unwired: 5 in, 2 out]
            n1884 = while {
              tunnel: w1902 -> [w1924]
              i -> [w1920]
              stop <- w1919 continue-if-true
              (unwired) TRUE ("line mode (F)")
              n1885 = Read from Text File "Read File"(file (use dialog)=w1924) -> (text=w1921:string)  [unwired: 3 in, 3 out]
              n1886 = local write "Numeric 11"(w1920) -> ()
              n1887 = String Length(string=w1921) -> (length=w1923:i32)
              n1888 = Greater?(x=w1923, y=1) -> (0:w1919:bool)
            }
            n1889 = while {
              tunnel: w1901 -> [w1930]
              i -> [w1926]
              stop <- w1925 continue-if-true
              (unwired) TRUE ("line mode (F)")
              n1890 = Read from Text File "Read File"(file (use dialog)=w1930) -> (text=w1927:string)  [unwired: 3 in, 3 out]
              n1891 = local write "Numeric 12"(w1926) -> ()
              n1892 = String Length(string=w1927) -> (length=w1929:i32)
              n1893 = Greater?(x=w1929, y=1) -> (0:w1925:bool)
            }
            n1894 = while {
              tunnel: w1900 -> [w1936]
              i -> [w1932]
              stop <- w1931 continue-if-true
              (unwired) TRUE ("line mode (F)")
              n1895 = Read from Text File "Read File"(file (use dialog)=w1936) -> (text=w1933:string)  [unwired: 3 in, 3 out]
              n1896 = local write "Numeric 13"(w1932) -> ()
              n1897 = String Length(string=w1933) -> (length=w1935:i32)
              n1898 = Greater?(x=w1935, y=1) -> (0:w1931:bool)
            }
            n1899 = String To Path(string=w1899) -> (path=w1907:path)
            n1900 = Open/Create/Replace File "Open File"(file path (use dialog)=w1907) -> (refnum out=w1903:refnum<file>)  [unwired: 5 in, 2 out]
            n1901 = while {
              tunnel: w1903 -> [w1918]
              i -> [w1914]
              stop <- w1913 continue-if-true
              (unwired) TRUE ("line mode (F)")
              n1902 = Read from Text File "Read File"(file (use dialog)=w1918) -> (text=w1915:string)  [unwired: 3 in, 3 out]
              n1903 = local write "Numeric 8"(w1914) -> ()
              n1904 = String Length(string=w1915) -> (length=w1917:i32)
              n1905 = Greater?(x=w1917, y=1) -> (0:w1913:bool)
            }
          }
          frame #1 {
            w2088 = FALSE ("ACTUAL   MERGE")
            # "Sample Temp"
            # "ECR"
            # "COF"
            # "Time\nCOF\nFF\nTemp"
            n1906 = case shown="True" w1961 {
              tunnel: [w2108 w2109] -> w1962
              frame False {
                n1907 = local read "string1"() -> (w2108:string)
              }
              frame True {
                n1908 = local read "String Indicator 4"() -> (w2109:string)
              }
            }
            n1909 = local read "string1 3"() -> (w2006:string)
            n1910 = String To Path(string=w1962) -> (path=w2093:path)
            n1911 = String To Path(string=w2006) -> (path=w2104:path)
            n1912 = local read "Numeric 12"() -> (w2090:i32)
            n1913 = local read "Numeric 8"() -> (w2092:i32)
            n1914 = local read "string1 2"() -> (w2007:string)
            n1915 = local read "string1 4"() -> (w2005:string)
            n1916 = Open/Create/Replace File "Open File"(file path (use dialog)=w2093) -> (refnum out=w2107:refnum<file>, error out=w2106:errorcluster)  [unwired: 5 in, 1 out]
            n1917 = Open/Create/Replace File "Open File"(file path (use dialog)=w2104) -> (refnum out=w2100:refnum<file>, error out=w2101:errorcluster)  [unwired: 5 in, 1 out]
            n1918 = for {
              N: w2092 -> [_]
              tunnel: w2107 -> [w2255]
              tunnel: w2106 -> [w2254]
              tunnel: [w2244] -> w2019 mode=indexing
              tunnel: [w2242] -> w2076 mode=indexing
              tunnel: [w2243] -> w2071 mode=indexing
              tunnel: w2088 -> [_]
              tunnel: [w2236] -> w2073 mode=indexing
              tunnel: [w2232] -> w2042 mode=indexing
              tunnel: [w2228] -> w2017 mode=indexing
              tunnel: [w2224] -> w1998 mode=indexing
              tunnel: [w2219] -> w1958 mode=indexing
              (unwired) TRUE ("line mode (F)")
              # "freq"
              # "Stroke"
              # "Time"
              # "CoF"
              # "Humidity"
              # "Temp"
              # "Air Temp"
              # "ECR"
              n1919 = Read from Text File "Read File"(file (use dialog)=w2255, error in=w2254) -> (text=w2220:string)  [unwired: 2 in, 3 out]
              n1920 = local write "String 6"(w2220) -> ()
              n1921 = String Subset(string=w2220, offset (0)=0, length (rest)=14 ("length (rest)")) -> (substring=w2248:string)
              n1922 = String Subset(string=w2220, offset (0)=35, length (rest)=9 ("length (rest)")) -> (substring=w2245:string)
              n1923 = String Subset(string=w2220, offset (0)=15, length (rest)=9 ("length (rest)")) -> (substring=w2251:string)
              n1924 = Fract/Exp String To Number(string=w2248) -> (number=w2244:dbl)  [unwired: 3 in, 1 out]
              n1925 = Fract/Exp String To Number(string=w2245) -> (number=w2243:dbl)  [unwired: 3 in, 1 out]
              n1926 = Fract/Exp String To Number(string=w2251) -> (number=w2242:dbl)  [unwired: 3 in, 1 out]
              n1927 = String Subset(string=w2220, offset (0)=85, length (rest)=9 ("length (rest)")) -> (substring=w2221:string)
              n1928 = String Subset(string=w2220, offset (0)=25, length (rest)=9 ("length (rest)")) -> (substring=w2227:string)
              n1929 = String Subset(string=w2220, offset (0)=55, length (rest)=9 ("length (rest)")) -> (substring=w2229:string)
              n1930 = String Subset(string=w2220, offset (0)=45, length (rest)=9 ("length (rest)")) -> (substring=w2235:string)
              n1931 = String Subset(string=w2220, offset (0)=65, length (rest)=9 ("length (rest)")) -> (substring=w2241:string)
              n1932 = Fract/Exp String To Number(string=w2227) -> (number=w2224:dbl)  [unwired: 3 in, 1 out]
              n1933 = Fract/Exp String To Number(string=w2221) -> (number=w2219:dbl)  [unwired: 3 in, 1 out]
              n1934 = Fract/Exp String To Number(string=w2229) -> (number=w2228:dbl)  [unwired: 3 in, 1 out]
              n1935 = Fract/Exp String To Number(string=w2235) -> (number=w2232:dbl)  [unwired: 3 in, 1 out]
              n1936 = Fract/Exp String To Number(string=w2241) -> (number=w2238:dbl)  [unwired: 3 in, 1 out]
              n1937 = Add(x=w2238, y=0.0) -> (x+y=w2236:dbl)
            }
            n1938 = for {
              N: w2090 -> [_]
              tunnel: w2101 -> [w2181]
              tunnel: w2100 -> [w2180]
              tunnel: [w2170] -> w2059 mode=indexing
              tunnel: [w2168] -> w2057 mode=indexing
              tunnel: [w2169] -> w2053 mode=indexing
              tunnel: w2088 -> [_]
              tunnel: [w2162] -> w2055 mode=indexing
              tunnel: [w2158] -> w2037 mode=indexing
              tunnel: [w2154] -> w2013 mode=indexing
              tunnel: [w2151] -> w1994 mode=indexing
              tunnel: [w2147] -> w1953 mode=indexing
              (unwired) 9 ("length (rest)")
              (unwired) 9 ("length (rest)")
              (unwired) TRUE ("line mode (F)")
              n1939 = Read from Text File "Read File"(file (use dialog)=w2180, error in=w2181) -> (text=w2148:string)  [unwired: 2 in, 3 out]
              n1940 = local write "String 8"(w2148) -> ()
              n1941 = String Subset(string=w2148, offset (0)=85) -> (substring=w2150:string)  [unwired: 1 in]
              n1942 = String Subset(string=w2148, offset (0)=35, length (rest)=9 ("length (rest)")) -> (substring=w2171:string)
              n1943 = String Subset(string=w2148, offset (0)=55, length (rest)=9 ("length (rest)")) -> (substring=w2156:string)
              n1944 = String Subset(string=w2148, offset (0)=25) -> (substring=w2152:string)  [unwired: 1 in]
              n1945 = String Subset(string=w2148, offset (0)=15, length (rest)=9 ("length (rest)")) -> (substring=w2177:string)
              n1946 = String Subset(string=w2148, offset (0)=0, length (rest)=14 ("length (rest)")) -> (substring=w2174:string)
              n1947 = String Subset(string=w2148, offset (0)=45, length (rest)=9 ("length (rest)")) -> (substring=w2161:string)
              n1948 = String Subset(string=w2148, offset (0)=65, length (rest)=9 ("length (rest)")) -> (substring=w2167:string)
              n1949 = Fract/Exp String To Number(string=w2150) -> (number=w2147:dbl)  [unwired: 3 in, 1 out]
              n1950 = Fract/Exp String To Number(string=w2171) -> (number=w2169:dbl)  [unwired: 3 in, 1 out]
              n1951 = Fract/Exp String To Number(string=w2156) -> (number=w2154:dbl)  [unwired: 3 in, 1 out]
              n1952 = Fract/Exp String To Number(string=w2152) -> (number=w2151:dbl)  [unwired: 3 in, 1 out]
              n1953 = Fract/Exp String To Number(string=w2177) -> (number=w2168:dbl)  [unwired: 3 in, 1 out]
              n1954 = Fract/Exp String To Number(string=w2174) -> (number=w2170:dbl)  [unwired: 3 in, 1 out]
              n1955 = Fract/Exp String To Number(string=w2161) -> (number=w2158:dbl)  [unwired: 3 in, 1 out]
              n1956 = Fract/Exp String To Number(string=w2167) -> (number=w2164:dbl)  [unwired: 3 in, 1 out]
              n1957 = Add(x=w2164, y=0.0) -> (x+y=w2162:dbl)
            }
            n1958 = String To Path(string=w2007) -> (path=w2105:path)
            n1959 = String To Path(string=w2005) -> (path=w2099:path)
            n1960 = local read "Numeric 11"() -> (w2089:i32)
            n1961 = local read "Numeric 13"() -> (w2091:i32)
            n1962 = Open/Create/Replace File "Open File"(file path (use dialog)=w2105) -> (refnum out=w2103:refnum<file>, error out=w2102:errorcluster)  [unwired: 5 in, 1 out]
            n1963 = Open/Create/Replace File "Open File"(file path (use dialog)=w2099) -> (refnum out=w2098:refnum<file>, error out=w2097:errorcluster)  [unwired: 5 in, 1 out]
            n1964 = for {
              N: w2089 -> [_]
              tunnel: w2103 -> [w2218]
              tunnel: w2102 -> [w2217]
              tunnel: [w2207] -> w2069 mode=indexing
              tunnel: [w2205] -> w2067 mode=indexing
              tunnel: [w2206] -> w2062 mode=indexing
              tunnel: w2088 -> [_]
              tunnel: [w2199] -> w2064 mode=indexing
              tunnel: [w2195] -> w2040 mode=indexing
              tunnel: [w2191] -> w2015 mode=indexing
              tunnel: [w2187] -> w1996 mode=indexing
              tunnel: [w2182] -> w1954 mode=indexing
              (unwired) TRUE ("line mode (F)")
              n1965 = Read from Text File "Read File"(file (use dialog)=w2218, error in=w2217) -> (text=w2183:string)  [unwired: 2 in, 3 out]
              n1966 = local write "String 7"(w2183) -> ()
              n1967 = String Subset(string=w2183, offset (0)=85, length (rest)=9 ("length (rest)")) -> (substring=w2186:string)
              n1968 = String Subset(string=w2183, offset (0)=35, length (rest)=9 ("length (rest)")) -> (substring=w2208:string)
              n1969 = String Subset(string=w2183, offset (0)=55, length (rest)=9 ("length (rest)")) -> (substring=w2194:string)
              n1970 = String Subset(string=w2183, offset (0)=25, length (rest)=9 ("length (rest)")) -> (substring=w2188:string)
              n1971 = String Subset(string=w2183, offset (0)=45, length (rest)=9 ("length (rest)")) -> (substring=w2196:string)
              n1972 = String Subset(string=w2183, offset (0)=0, length (rest)=14 ("length (rest)")) -> (substring=w2211:string)
              n1973 = String Subset(string=w2183, offset (0)=15, length (rest)=9 ("length (rest)")) -> (substring=w2214:string)
              n1974 = String Subset(string=w2183, offset (0)=65, length (rest)=9 ("length (rest)")) -> (substring=w2200:string)
              n1975 = Fract/Exp String To Number(string=w2186) -> (number=w2182:dbl)  [unwired: 3 in, 1 out]
              n1976 = Fract/Exp String To Number(string=w2208) -> (number=w2206:dbl)  [unwired: 3 in, 1 out]
              n1977 = Fract/Exp String To Number(string=w2194) -> (number=w2191:dbl)  [unwired: 3 in, 1 out]
              n1978 = Fract/Exp String To Number(string=w2188) -> (number=w2187:dbl)  [unwired: 3 in, 1 out]
              n1979 = Fract/Exp String To Number(string=w2196) -> (number=w2195:dbl)  [unwired: 3 in, 1 out]
              n1980 = Fract/Exp String To Number(string=w2211) -> (number=w2207:dbl)  [unwired: 3 in, 1 out]
              n1981 = Fract/Exp String To Number(string=w2214) -> (number=w2205:dbl)  [unwired: 3 in, 1 out]
              n1982 = Fract/Exp String To Number(string=w2200) -> (number=w2203:dbl)  [unwired: 3 in, 1 out]
              n1983 = Add(x=w2203, y=0.0) -> (x+y=w2199:dbl)
            }
            n1984 = for {
              N: w2091 -> [_]
              tunnel: w2098 -> [w2146]
              tunnel: w2097 -> [w2145]
              tunnel: [w2135] -> w2051 mode=indexing
              tunnel: [w2134] -> w2044 mode=indexing
              tunnel: w2088 -> [_]
              tunnel: [w2123] -> w2049 mode=indexing
              tunnel: [w2128] -> w2046 mode=indexing
              tunnel: [w2124] -> w2036 mode=indexing
              tunnel: [w2119] -> w2011 mode=indexing
              tunnel: [w2115] -> w1992 mode=indexing
              tunnel: [w2110] -> w1952 mode=indexing
              (unwired) 1.0 ("x")
              (unwired) TRUE ("line mode (F)")
              n1985 = Read from Text File "Read File"(file (use dialog)=w2146, error in=w2145) -> (text=w2111:string)  [unwired: 2 in, 3 out]
              n1986 = local write "String 12"(w2111) -> ()
              n1987 = String Subset(string=w2111, offset (0)=85, length (rest)=9 ("length (rest)")) -> (substring=w2113:string)
              n1988 = String Subset(string=w2111, offset (0)=35, length (rest)=9 ("length (rest)")) -> (substring=w2136:string)
              n1989 = String Subset(string=w2111, offset (0)=55, length (rest)=9 ("length (rest)")) -> (substring=w2121:string)
              n1990 = String Subset(string=w2111, offset (0)=25, length (rest)=9 ("length (rest)")) -> (substring=w2117:string)
              n1991 = String Subset(string=w2111, offset (0)=45, length (rest)=9 ("length (rest)")) -> (substring=w2126:string)
              n1992 = String Subset(string=w2111, offset (0)=15, length (rest)=9 ("length (rest)")) -> (substring=w2142:string)
              n1993 = String Subset(string=w2111, offset (0)=0, length (rest)=14 ("length (rest)")) -> (substring=w2139:string)
              n1994 = String Subset(string=w2111, offset (0)=65, length (rest)=9 ("length (rest)")) -> (substring=w2129:string)
              n1995 = Fract/Exp String To Number(string=w2113) -> (number=w2110:dbl)  [unwired: 3 in, 1 out]
              n1996 = Fract/Exp String To Number(string=w2136) -> (number=w2134:dbl)  [unwired: 3 in, 1 out]
              n1997 = Fract/Exp String To Number(string=w2121) -> (number=w2119:dbl)  [unwired: 3 in, 1 out]
              n1998 = Fract/Exp String To Number(string=w2117) -> (number=w2115:dbl)  [unwired: 3 in, 1 out]
              n1999 = Fract/Exp String To Number(string=w2126) -> (number=w2124:dbl)  [unwired: 3 in, 1 out]
              n2000 = Fract/Exp String To Number(string=w2142) -> (number=w2123:dbl)  [unwired: 3 in, 1 out]
              n2001 = Fract/Exp String To Number(string=w2139) -> (number=w2135:dbl)  [unwired: 3 in, 1 out]
              n2002 = Fract/Exp String To Number(string=w2129) -> (number=w2132:dbl)  [unwired: 3 in, 1 out]
              n2003 = Add(x=w2132, y=0.0) -> (x+y=w2128:dbl)
            }
            n2004 = Delete From Array(array=w1994, index=0) -> (array with subset deleted=w1967:dbl[])  [unwired: 1 in, 1 out]
            n2005 = Delete From Array(array=w2057, index=0) -> (array with subset deleted=w2030:dbl[])  [unwired: 1 in, 1 out]
            n2006 = Delete From Array(array=w2037, index=0) -> (array with subset deleted=w2025:dbl[])  [unwired: 1 in, 1 out]
            n2007 = Delete From Array(array=w2055, index=0) -> (array with subset deleted=w2056:dbl[])  [unwired: 1 in, 1 out]
            n2008 = call-poly <vilib>:"Mean.vi"("X"=w1967) -> ("mean"=→"КОФ2 4":dbl)  [unwired: 1 out]
            n2009 = call-poly <vilib>:"Mean.vi"("X"=w2030) -> ("mean"=→"КОФ3":dbl)  [unwired: 1 out]
            n2010 = call-poly <vilib>:"Mean.vi"("X"=w2025) -> ("mean"=→"CP3":dbl)  [unwired: 1 out]
            n2011 = Delete From Array(array=w2019, index=0) -> (array with subset deleted=w1946:dbl[])  [unwired: 1 in, 1 out]
            n2012 = Delete From Array(array=w1958, index=0) -> (array with subset deleted=w1945:dbl[])  [unwired: 1 in, 1 out]
            n2013 = Delete From Array(array=w1998, index=0) -> (array with subset deleted=w1969:dbl[])  [unwired: 1 in, 1 out]
            n2014 = Delete From Array(array=w2076, index=0) -> (array with subset deleted=w2031:dbl[])  [unwired: 1 in, 1 out]
            n2015 = Delete From Array(array=w2042, index=0) -> (array with subset deleted=w2027:dbl[])  [unwired: 1 in, 1 out]
            "array w/ subset deleted" <- w2027
            n2016 = Delete From Array(array=w2073, index=0) -> (array with subset deleted=w2074:dbl[])  [unwired: 1 in, 1 out]
            n2017 = call-poly <vilib>:"Mean.vi"("X"=w1969) -> ("mean"=→"КОФ2 2":dbl)  [unwired: 1 out]
            n2018 = call-poly <vilib>:"Mean.vi"("X"=w2031) -> ("mean"=→"КОФ1":dbl)  [unwired: 1 out]
            n2019 = Bundle "Bundle"(w1946, w1945) -> (w1951:cluster{dbl[], dbl[]})  [unwired: 1 in]
            n2020 = Bundle "Bundle"(w1946, w2074) -> (w1938:cluster{dbl[], dbl[]})  [unwired: 1 in]
            n2021 = Delete From Array(array=w1953, index=0) -> (array with subset deleted=w1941:dbl[])  [unwired: 1 in, 1 out]
            n2022 = Delete From Array(array=w1954, index=0) -> (array with subset deleted=w1943:dbl[])  [unwired: 1 in, 1 out]
            n2023 = Delete From Array(array=w2064, index=0) -> (array with subset deleted=w2065:dbl[])  [unwired: 1 in, 1 out]
            n2024 = Delete From Array(array=w1952, index=0) -> (array with subset deleted=w1939:dbl[])  [unwired: 1 in, 1 out]
            n2025 = Delete From Array(array=w2046, index=0) -> (array with subset deleted=w2047:dbl[])  [unwired: 1 in, 1 out]
            n2026 = Delete From Array(array=w2071, index=0) -> (array with subset deleted=w1977:dbl[])  [unwired: 1 in, 1 out]
            n2027 = Delete From Array(array=w2017, index=0) -> (array with subset deleted=w1973:dbl[])  [unwired: 1 in, 1 out]
            n2028 = Delete From Array(array=w2053, index=0) -> (array with subset deleted=w1975:dbl[])  [unwired: 1 in, 1 out]
            n2029 = Delete From Array(array=w2013, index=0) -> (array with subset deleted=w1971:dbl[])  [unwired: 1 in, 1 out]
            n2030 = Delete From Array(array=w2062, index=0) -> (array with subset deleted=w1976:dbl[])  [unwired: 1 in, 1 out]
            n2031 = Delete From Array(array=w2015, index=0) -> (array with subset deleted=w1972:dbl[])  [unwired: 1 in, 1 out]
            n2032 = Delete From Array(array=w1996, index=0) -> (array with subset deleted=w1968:dbl[])  [unwired: 1 in, 1 out]
            n2033 = Delete From Array(array=w2040, index=0) -> (array with subset deleted=w2026:dbl[])  [unwired: 1 in, 1 out]
            n2034 = Delete From Array(array=w2067, index=0) -> (array with subset deleted=w2028:dbl[])  [unwired: 1 in, 1 out]
            n2035 = Delete From Array(array=w2044, index=0) -> (array with subset deleted=w1974:dbl[])  [unwired: 1 in, 1 out]
            n2036 = Delete From Array(array=w2011, index=0) -> (array with subset deleted=w1970:dbl[])  [unwired: 1 in, 1 out]
            n2037 = Delete From Array(array=w1992, index=0) -> (array with subset deleted=w1966:dbl[])  [unwired: 1 in, 1 out]
            n2038 = Delete From Array(array=w2036, index=0) -> (array with subset deleted=w2024:dbl[])  [unwired: 1 in, 1 out]
            n2039 = Delete From Array(array=w2049, index=0) -> (array with subset deleted=w2029:dbl[])  [unwired: 1 in, 1 out]
            n2040 = Delete From Array(array=w2059, index=0) -> (array with subset deleted=w1942:dbl[])  [unwired: 1 in, 1 out]
            n2041 = Delete From Array(array=w2069, index=0) -> (array with subset deleted=w1944:dbl[])  [unwired: 1 in, 1 out]
            n2042 = Delete From Array(array=w2051, index=0) -> (array with subset deleted=w1940:dbl[])  [unwired: 1 in, 1 out]
            n2043 = Bundle "Bundle"(w1946, w1977) -> (w1964:cluster{dbl[], dbl[]})  [unwired: 1 in]
